vi "Execute Command On Target.vi"(8 "error in (no error)":errorcluster, 11 "Session in":refnum<class "Session.lvclass">) -> (0 "error out":errorcluster, 1 "Status":T2, 2 "Output":string, 3 "Session out":refnum<class "Session.lvclass">, 4 "Errors":T1[](array[typedef]))   [LabVIEW 2015, in "WinSCP.lvlib" / "Session.lvclass"]
uses:
  Session.lvclass
  CommandExecution/Status.ctl
  CommandExecution/ErrorDescription.ctl
  CommandExecution/Command Execution.lvclass
  Session.lvclass/Session.ctl
panel:
  in  "Command":string
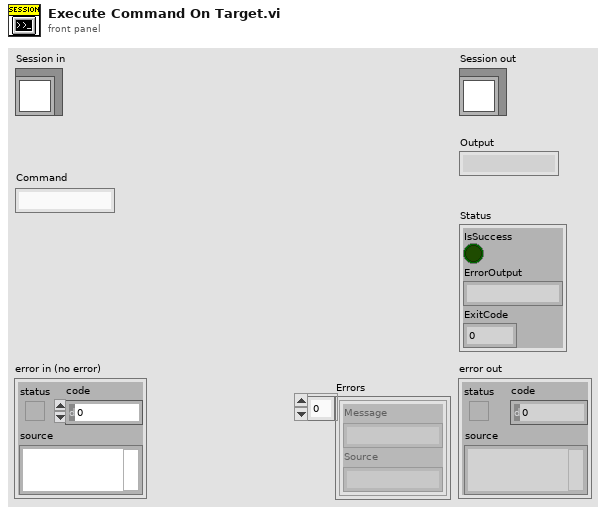
[diagram p1: front panel]
types:
  T1 = typedef "WinSCP.lvlib/Command Execution.lvclass/ErrorDescription.ctl" = cluster{"Message":string, "Source":string}
  T2 = typedef "WinSCP.lvlib/Command Execution.lvclass/Status.ctl" = cluster{"IsSuccess":bool, "ErrorOutput":string, "ExitCode":i32}
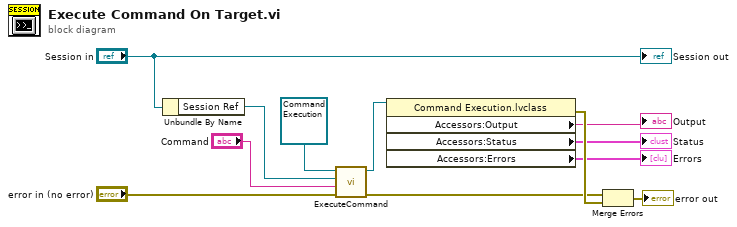
[diagram p0: block diagram]
diagram:
  n1 = Unbundle By Name("Session in") -> ("Session Ref"=w6:refnum<k24>)
  n2 = call-dynamic "ExecuteCommand.vi"("error in"="error in (no error)", "Command"="Command", "Session Ref"=w6, "Command Execution in"=refnum<class "Command Execution.lvclass"> refnum) -> ("error out"=w9:errorcluster, "Command Execution out"=w5:refnum<class "Command Execution.lvclass">)  [unwired: 6 in]
  n3 = property class="Command Execution.lvclass"(reference=w5) -> (error out=w12:errorcluster, "Accessors:Output"=→"Output":string, "Accessors:Status"=→"Status":T2, "Accessors:Errors"=→"Errors":T1[])  [unwired: 1 in, 1 out]
  n4 = Merge Errors(w9, w12) -> (→"error out":errorcluster)
  "Session out" <- "Session in"
